vi "Read Humidity DBL.vi"(8 "error in":errorcluster, 10 "Source":string, 11 "IRead Absolute Humidity in":refnum<class "IRead Humidity.lvclass">) -> (0 "error out":errorcluster, 1 "Time Stamp":timestamp format="%<%x %.3X>T", 2 "Humidity":dbl, 3 "IRead Absolute Humidity out":refnum<class "IRead Humidity.lvclass">)   [LabVIEW 2024, in "IRead Humidity.lvclass"]
uses:
  IRead Humidity.lvclass
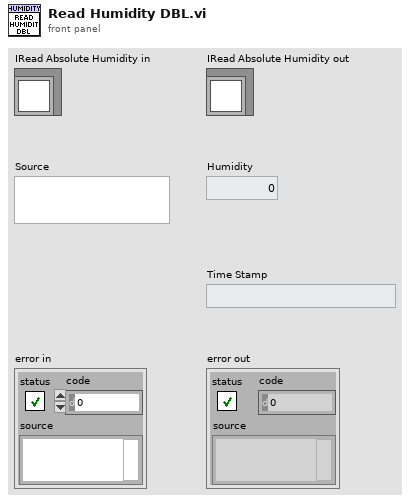
[diagram p1: front panel]
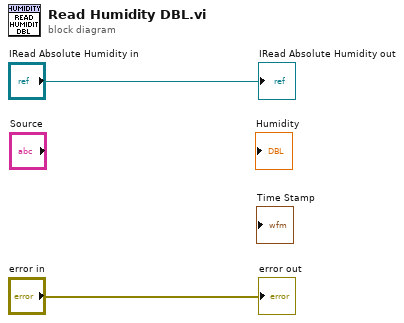
[diagram p0: block diagram]
diagram:
  "error out" <- "error in"
  "IRead Absolute Humidity out" <- "IRead Absolute Humidity in"
